vi "Scene func global.vi"(4 "Face of interest":u8, 6 "Angle":sgl, 7 "Axis":cluster{"X":sgl, "Y":sgl, "Z":sgl}, 8 "error in (no error)":errorcluster, 9 "Facets To move":T1[](array[typedef]), 10 "Rubix Text Array":string[][](array[string]), 11 "Commands":T2=enum."Generate Rubix Array") -> (0 "error out":errorcluster, 1 "Rubix ref Array":refnum<vi>[][](array[refnum]))   [LabVIEW 2019]
uses:
  Scene Commands.ctl
  Rubix Array data type.ctl
  scene func global data.ctl
  <vilib>/Utility/miscctls.llb/LVRectTypeDef.ctl
  <vilib>/picture/3D Picture Control/Object/Create Object (name).vi
  <vilib>/picture/3D Picture Control/NI_3D Picture Control.lvlib
panel:
  out "Rubix Array 2":T1[][](array[typedef])
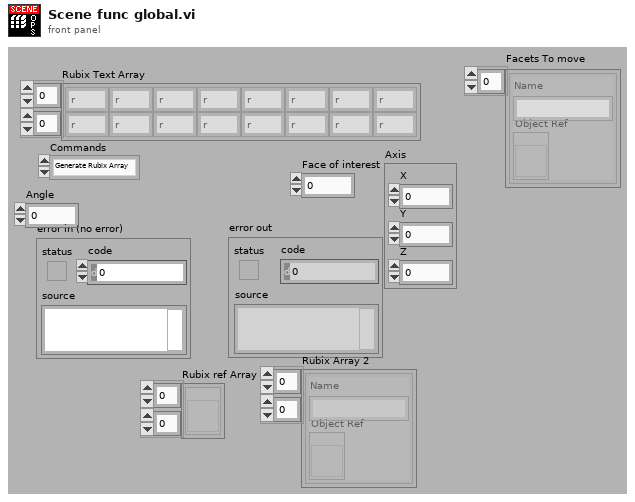
[diagram p1: front panel]
types:
  T1 = typedef "Rubix Array data type.ctl" = cluster{"Object Ref":refnum<vi>, "Name":string}
  T2 = typedef "Scene Commands.ctl" = enum16{"Init", "Set Rubix Text Array", "Get Rubix Ref Array", "Generate Rubix Array", "Get Rubix Array", "Show Render Window", "Go To Face", "Rotate", "Update Scene", "Clear Rubix"}
  T3 = enum16{"Open", "Minimized", "Maximized", "Hidden"}
  T4 = typedef "scene func global data.ctl" = cluster{"Rubix Text Array":string[][], "Scene:New Object":refnum<vi>, "error out":errorcluster, "New Window Refnum":refnum<vi>, "Camera Position":cluster{"X":sgl, "Y":sgl, "Z":sgl}, "Rubix ref Array ":refnum<vi>[][], "Rubix Array":T1[][]}
  T5 = typedef "LVRectTypeDef.ctl" = cluster{"Left":i16, "Top":i16, "Right":i16, "Bottom":i16}
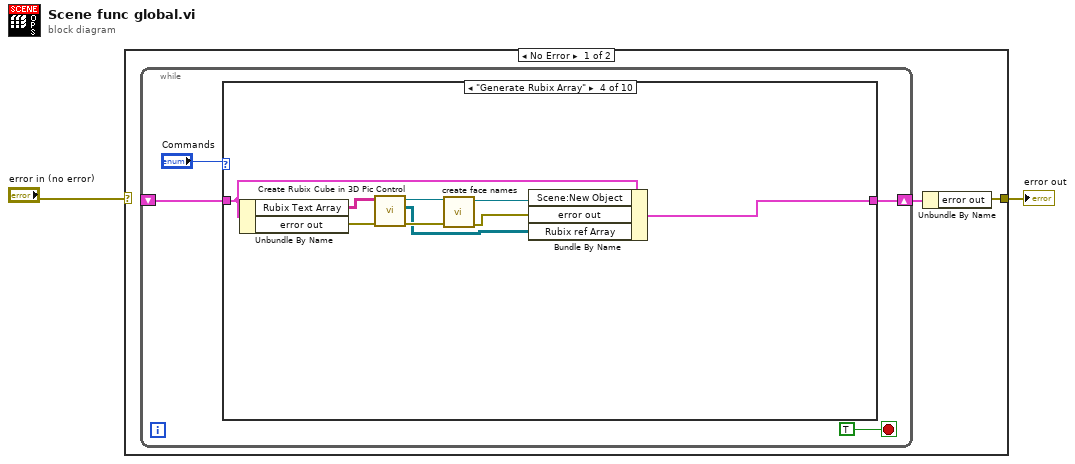
[diagram p0: block diagram]
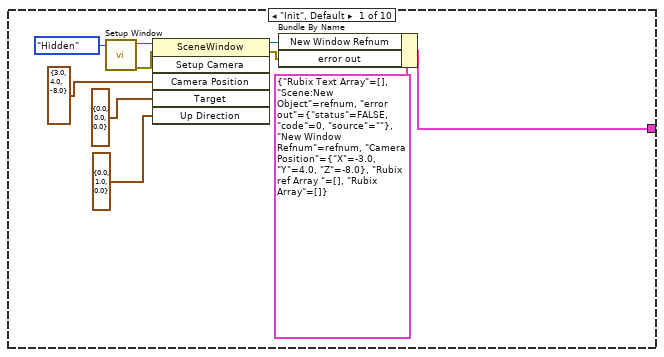
[diagram p2: hidden frame]
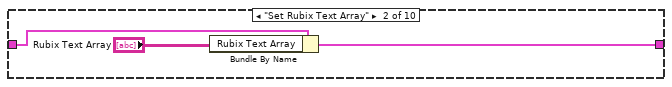
[diagram p3: hidden frame]
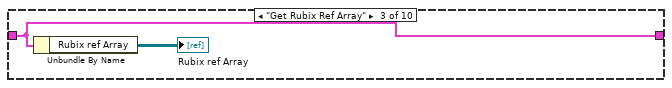
[diagram p4: hidden frame]
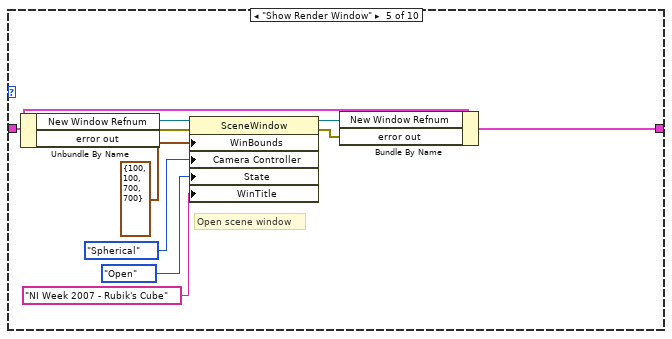
[diagram p5: hidden frame]
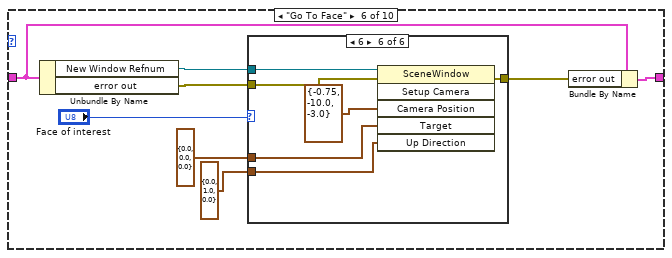
[diagram p6: hidden frame]
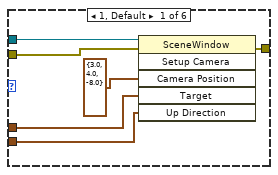
[diagram p7: hidden frame]
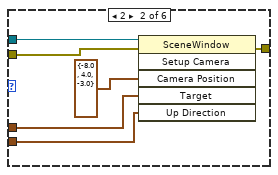
[diagram p8: hidden frame]
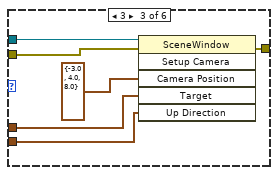
[diagram p9: hidden frame]
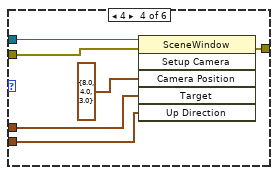
[diagram p10: hidden frame]
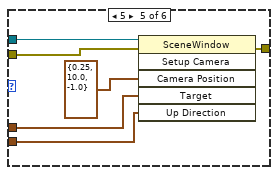
[diagram p11: hidden frame]
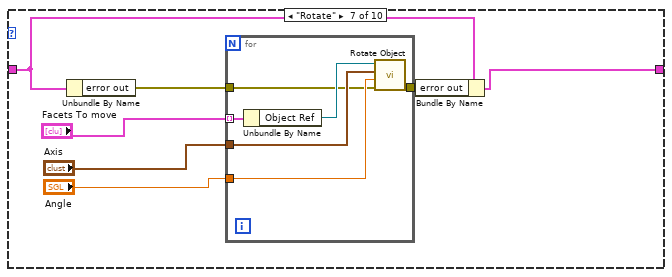
[diagram p12: hidden frame]
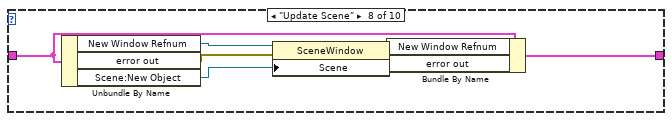
[diagram p13: hidden frame]
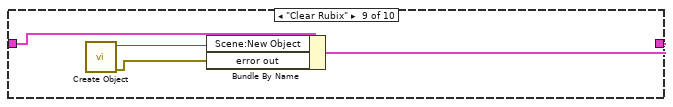
[diagram p14: hidden frame]
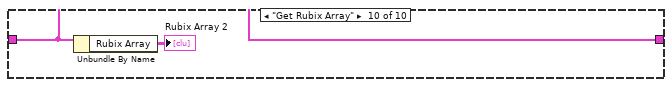
[diagram p15: hidden frame]
diagram:
  n1 = case shown="No Error" "error in (no error)" {
    selector: "error in (no error)" -> [_ w113]
    tunnel: [w3 w113] -> w1
    frame No Error {
      n2 = while {
        shift-right: [w6] -> w4
        shift-left: _ -> [w5]
        stop <- TRUE stop-if-true
        n3 = case shown="\"Generate Rubix Array\"" "Commands" {
          tunnel: [w17 w20 w23 w31 w42 w44 w88 w105 w108 w111] -> w6
          tunnel: w5 -> [_ w19 w23 w32 w37 w45 w90 w106 w110 w111]
          frame "Init", Default {
            n4 = call <vilib>:"Setup Window.vi"("Window State"=T3."Hidden") -> ("error out"=w13:errorcluster, "New Window Refnum"=w9:refnum<vi>)  [unwired: 9 in]
            n5 = invoke class="SceneWindow" method="Setup Camera"(reference=w9, error in=w13, "Camera Position"=cluster{"X":sgl, "Y":sgl, "Z":sgl} {"X"=3.0, "Y"=4.0, "Z"=-8.0}, "Target"=cluster{"X":sgl, "Y":sgl, "Z":sgl} {"X"=0.0, "Y"=0.0, "Z"=0.0}, "Up Direction"=cluster{"X":sgl, "Y":sgl, "Z":sgl} {"X"=0.0, "Y"=1.0, "Z"=0.0}) -> (reference out=w15:refnum<vi>, error out=w14:errorcluster)  [unwired: 1 in, 4 out]
            n6 = Bundle By Name(cluster=T4 {"Rubix Text Array"=[], "Scene:New Object"=refnum, "error out"={"status"=FALSE, "code"=0, "source"=""}, "New Window Refnum"=refnum, "Camera Position"={"X"=-3.0, "Y"=4.0, "Z"=-8.0}, "Rubix ref Array "=[], "Rubix Array"=[]} ("output cluster"), "New Window Refnum"=w15, "error out"=w14) -> (w17:T4)
          }
          frame "Set Rubix Text Array" {
            n7 = Bundle By Name(cluster=w19, "Rubix Text Array"="Rubix Text Array") -> (w20:T4)
          }
          frame "Get Rubix Ref Array" {
            n8 = Unbundle By Name(w23) -> ("Rubix ref Array"=→"Rubix ref Array":refnum<vi>[][])
          }
          frame "Generate Rubix Array" {
            n9 = Unbundle By Name(w32) -> ("Rubix Text Array"=w24:string[][], "error out"=w26:errorcluster)
            n10 = call "Create Rubix Cube in 3D Pic Control.vi"("error in (no error)"=w26, "RubixTab solver"=w24) -> ("error out"=w28:errorcluster, "Rubix Array"=w25:refnum<vi>[][], "Scene:New Object"=w30:refnum<vi>)  [unwired: 7 in]
            n11 = call "create face names.vi"("error out 2"=w28, "Scene:New Object 2"=w30) -> ("error out"=w27:errorcluster, "Scene:New Object"=w29:refnum<vi>)  [unwired: 8 in]
            n12 = Bundle By Name(cluster=w32, "Scene:New Object"=w29, "error out"=w27, "Rubix ref Array"=w25) -> (w31:T4)
          }
          frame "Show Render Window" {
            # "Open scene window"
            n13 = Unbundle By Name(w37) -> ("New Window Refnum"=w36:refnum<vi>, "error out"=w34:errorcluster)
            n14 = property class="SceneWindow"(reference=w36, error in=w34, "WinBounds"=T5 {"Left"=100, "Top"=100, "Right"=700, "Bottom"=700} ("Window Bounds"), "Camera Controller"=enum16{"None", "Spherical", "Flying"}."Spherical" ("Camera Controller:Type"), "State"=T3."Open" ("Window State"), "WinTitle"="NI Week 2007 - Rubik's Cube" ("Window Title")) -> (reference out=w39:refnum<vi>, error out=w35:errorcluster)
            n15 = Bundle By Name(cluster=w37, "New Window Refnum"=w39, "error out"=w35) -> (w42:T4)
          }
          frame "Go To Face" {
            n16 = Unbundle By Name(w45) -> ("New Window Refnum"=w50:refnum<vi>, "error out"=w46:errorcluster)
            n17 = case shown="6" "Face of interest" {
              tunnel: w50 -> [w56 w62 w68 w74 w80 w86]
              tunnel: cluster{"X":sgl, "Y":sgl, "Z":sgl} {"X"=0.0, "Y"=0.0, "Z"=0.0} ("Target") -> [w55 w61 w67 w73 w79 w85]
              tunnel: cluster{"X":sgl, "Y":sgl, "Z":sgl} {"X"=0.0, "Y"=1.0, "Z"=0.0} ("Up Direction") -> [w54 w60 w66 w72 w78 w84]
              tunnel: w46 -> [w53 w59 w65 w71 w77 w83]
              tunnel: [w52 w58 w64 w70 w76 w82] -> w43
              frame 1, Default {
                n18 = invoke class="SceneWindow" method="Setup Camera"(reference=w56, error in=w53, "Camera Position"=cluster{"X":sgl, "Y":sgl, "Z":sgl} {"X"=3.0, "Y"=4.0, "Z"=-8.0}, "Target"=w55, "Up Direction"=w54) -> (error out=w52:errorcluster)  [unwired: 1 in, 5 out]
              }
              frame 2 {
                n19 = invoke class="SceneWindow" method="Setup Camera"(reference=w62, error in=w59, "Camera Position"=cluster{"X":sgl, "Y":sgl, "Z":sgl} {"X"=-8.0, "Y"=4.0, "Z"=-3.0}, "Target"=w61, "Up Direction"=w60) -> (error out=w58:errorcluster)  [unwired: 1 in, 5 out]
              }
              frame 3 {
                n20 = invoke class="SceneWindow" method="Setup Camera"(reference=w68, error in=w65, "Camera Position"=cluster{"X":sgl, "Y":sgl, "Z":sgl} {"X"=-3.0, "Y"=4.0, "Z"=8.0}, "Target"=w67, "Up Direction"=w66) -> (error out=w64:errorcluster)  [unwired: 1 in, 5 out]
              }
              frame 4 {
                n21 = invoke class="SceneWindow" method="Setup Camera"(reference=w74, error in=w71, "Camera Position"=cluster{"X":sgl, "Y":sgl, "Z":sgl} {"X"=8.0, "Y"=4.0, "Z"=3.0}, "Target"=w73, "Up Direction"=w72) -> (error out=w70:errorcluster)  [unwired: 1 in, 5 out]
              }
              frame 5 {
                n22 = invoke class="SceneWindow" method="Setup Camera"(reference=w80, error in=w77, "Camera Position"=cluster{"X":sgl, "Y":sgl, "Z":sgl} {"X"=0.25, "Y"=10.0, "Z"=-1.0}, "Target"=w79, "Up Direction"=w78) -> (error out=w76:errorcluster)  [unwired: 1 in, 5 out]
              }
              frame 6 {
                n23 = invoke class="SceneWindow" method="Setup Camera"(reference=w86, error in=w83, "Camera Position"=cluster{"X":sgl, "Y":sgl, "Z":sgl} {"X"=-0.75, "Y"=-10.0, "Z"=-3.0}, "Target"=w85, "Up Direction"=w84) -> (error out=w82:errorcluster)  [unwired: 1 in, 5 out]
              }
            }
            n24 = Bundle By Name(cluster=w45, "error out"=w43) -> (w44:T4)
          }
          frame "Rotate" {
            n25 = Unbundle By Name(w90) -> ("error out"=w91:errorcluster)
            n26 = for {
              tunnel: [w99] -> w89
              tunnel: "Axis" -> [w98]
              tunnel: "Angle" -> [w97]
              tunnel: w91 -> [w94]
              tunnel: "Facets To move" -> [w96] mode=indexing
              n27 = Unbundle By Name(w96) -> ("Object Ref"=w95:refnum<vi>)
              n28 = call <vilib>:"Rotate Object.vi"("error in (no error)"=w94, "Angle"=w97, "Axis"=w98, "Scene.Object In"=w95) -> ("error out"=w99:errorcluster)  [unwired: 6 in, 1 out]
            }
            n29 = Bundle By Name(cluster=w90, "error out"=w89) -> (w88:T4)
          }
          frame "Update Scene" {
            n30 = Unbundle By Name(w106) -> ("New Window Refnum"=w102:refnum<vi>, "error out"=w100:errorcluster, "Scene:New Object"=w101:refnum<vi>)
            n31 = property class="SceneWindow"(reference=w102, error in=w100, "Scene"=w101) -> (reference out=w104:refnum<vi>, error out=w103:errorcluster)
            n32 = Bundle By Name(cluster=w106, "New Window Refnum"=w104, "error out"=w103) -> (w105:T4)
          }
          frame "Clear Rubix" {
            n33 = call-poly <vilib>:"Create Object.vi"() -> ("error out"=w107:errorcluster, "Scene:New Object"=w109:refnum<vi>)  [unwired: 10 in]
            n34 = Bundle By Name(cluster=w110, "Scene:New Object"=w109, "error out"=w107) -> (w108:T4)
          }
          frame "Get Rubix Array" {
            n35 = Unbundle By Name(w111) -> ("Rubix Array"=→"Rubix Array 2":T1[][])
          }
        }
      }
      n36 = Unbundle By Name(w4) -> ("error out"=w3:errorcluster)
    }
    frame Error {
    }
  }
  "error out" <- w1
